vi "Lab02_LabViewArray&ForLoopP2_Bennett.vi"() -> ()   [LabVIEW 2017]
uses:
  <vilib>/Analysis/NI_AALBase.lvlib
panel:
  in  "stop":bool
  out "Std Dev":dbl
  out "Current Value":dbl
  out "Above Mean":bool
  out "Above Mean + Std Dev":bool
  in  "Wait Time":dbl
  out "Mean":dbl
  in  "Num List":dbl[](array[numeric])
  # "ELEC3800: IoT                      Lab02: Part II                      Matt Bennett\nFall 2017                                                                           09/12/17"
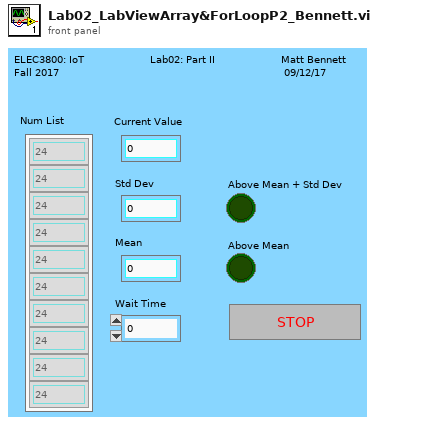
[diagram p1: front panel]
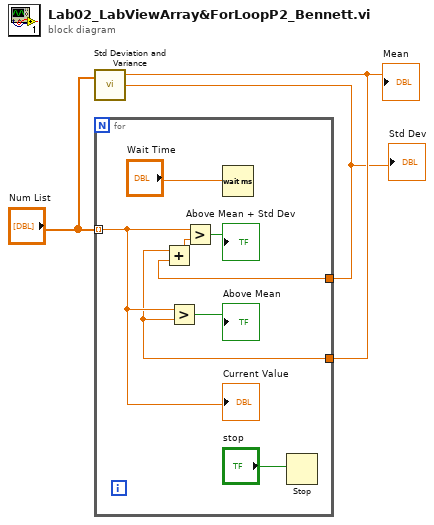
[diagram p0: block diagram]
diagram:
  n1 = call <vilib>:"Std Deviation and Variance.vi"("X"="Num List") -> ("mean"=w2:dbl, "standard deviation"=w1:dbl)  [unwired: 1 in, 1 out]
  "Mean" <- w2
  "Std Dev" <- w1
  n2 = for {
    tunnel: "Num List" -> [w8] mode=indexing
    tunnel: w1 -> [w7]
    tunnel: w2 -> [w5]
    n3 = Add(x=w5, y=w7) -> (x+y=w6:dbl)
    n4 = Greater?(x=w8, y=w5) -> (0:→"Above Mean":bool)
    n5 = Greater?(x=w8, y=w6) -> (0:→"Above Mean + Std Dev":bool)
    n6 = Wait (ms)(milliseconds to wait="Wait Time") -> ()  [unwired: 1 out]
    n7 = Stop(stop? (T)="stop") -> ()
    "Current Value" <- w8
  }
